vi "Set KH Coupling.vi"(8 "error in (no error)":errorcluster, 10 "Coupling":T1=enum."DC", 11 "KH Cluster":T2) -> (0 "error out":errorcluster, 3 "KH Cluster out":T2)   [LabVIEW 2016, in "Control Experiment UI.lvclass"]
uses:
  Control Experiment UI.lvclass
  Typedefs/KH Cluster--Cluster.ctl
  <userlib>/LevyLab/Krohn Hite 7008/typedefs/SetAll-Cluster.ctl
  <userlib>/LevyLab/Krohn Hite 7008/typedefs/Channel-Enum.ctl
  <userlib>/LevyLab/Krohn Hite 7008/typedefs/Gain-Enum.ctl
  <userlib>/LevyLab/Krohn Hite 7008/typedefs/Filter-Enum.ctl
  <userlib>/LevyLab/Krohn Hite 7008/typedefs/Shunt-Enum.ctl
  <userlib>/LevyLab/Krohn Hite 7008/typedefs/Coupling-Enum.ctl
  <userlib>/LevyLab/Krohn Hite 7008/typedefs/Input Configuration-Enum.ctl
  <userlib>/LevyLab/Krohn Hite 7008/Instrument.KH7008.lvclass
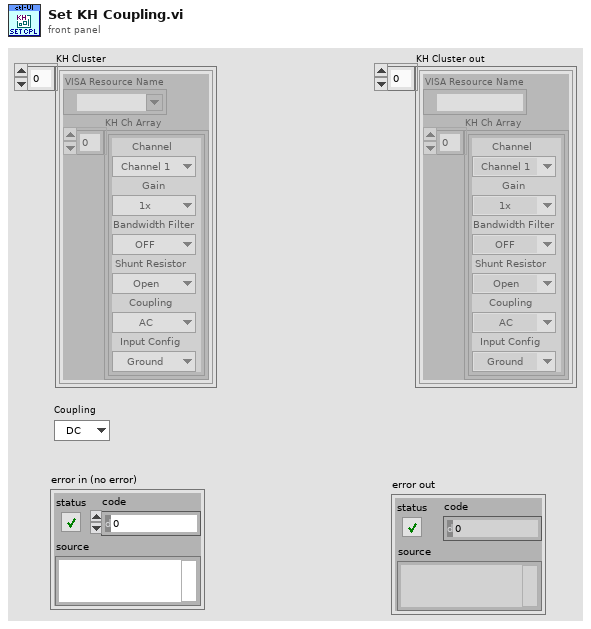
[diagram p1: front panel]
types:
  T1 = typedef "Instrument.KH7008.lvclass/Coupling-Enum.ctl" = enum16{"AC", "DC"}
  T2 = typedef "KH Cluster--Cluster.ctl" = cluster{"VISA Resource Name":refnum<visa-resource-name>, "KH Ch Array":T3[]}[]
  T3 = typedef "Instrument.KH7008.lvclass/SetAll-Cluster.ctl" = cluster{"Channel":T4, "Gain":T5, "Bandwidth Filter":T6, "Shunt Resistor":T7, "Coupling":T1, "Input Config":T8}
  T4 = typedef "Instrument.KH7008.lvclass/Channel-Enum.ctl" = enum16{"Channel 1", "Channel 2", "Channel 3", "Channel 4", "Channel 5", "Channel 6", "Channel 7", "Channel 8"}
  T5 = typedef "Instrument.KH7008.lvclass/Gain-Enum.ctl" = enum16{"1x", "10x", "100x", "1000x"}
  T6 = typedef "Instrument.KH7008.lvclass/Filter-Enum.ctl" = enum16{"OFF", "ON"}
  T7 = typedef "Instrument.KH7008.lvclass/Shunt-Enum.ctl" = enum16{"Open", "50 Ohms", "500 Ohms", "5k Ohms", "50k Ohms", "10M Ohm"}
  T8 = typedef "Instrument.KH7008.lvclass/Input Configuration-Enum.ctl" = enum16{"Ground", "SE+ (-gnd)", "SE- (+gnd)", "Differential"}
  T9 = cluster{"VISA Resource Name":refnum<visa-resource-name>, "KH Ch Array":T3[]}
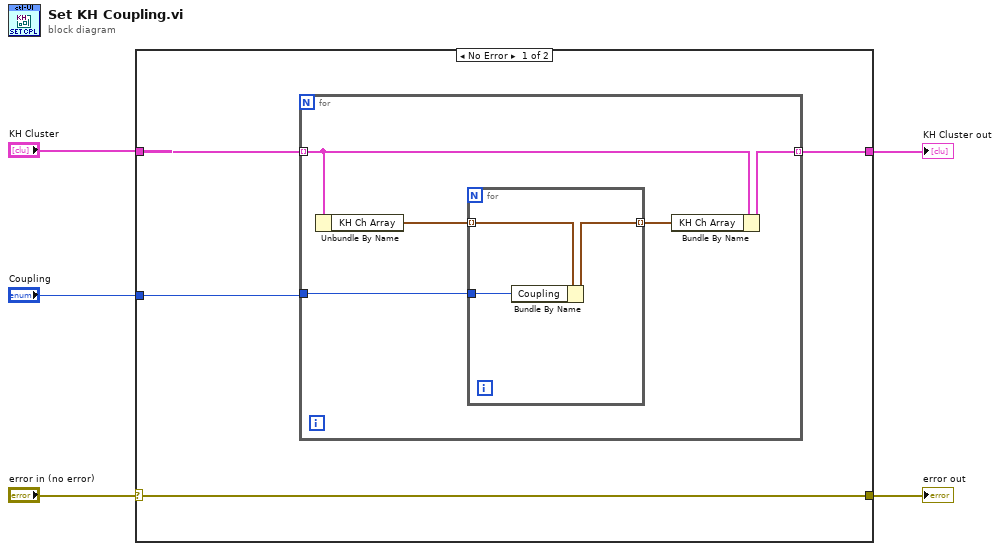
[diagram p0: block diagram]
diagram:
  n1 = case shown="No Error" "error in (no error)" {
    selector: "error in (no error)" -> [w8 w18]
    tunnel: "Coupling" -> [w6 _]
    tunnel: "KH Cluster" -> [w9 w19]
    tunnel: [w8 w18] -> w1
    tunnel: [w7 w19] -> w2
    frame No Error {
      n2 = for {
        tunnel: w9 -> [w14] mode=indexing
        tunnel: [w13] -> w7 mode=indexing
        tunnel: w6 -> [w10]
        n3 = Unbundle By Name(w14) -> ("KH Ch Array"=w12:T3[])
        n4 = for {
          tunnel: w12 -> [w17] mode=indexing
          tunnel: [w16] -> w11 mode=indexing
          tunnel: w10 -> [w15]
          n5 = Bundle By Name(cluster=w17, "Coupling"=w15) -> (w16:T3)
        }
        n6 = Bundle By Name(cluster=w14, "KH Ch Array"=w11) -> (w13:T9)
      }
    }
    frame Error {
    }
  }
  "KH Cluster out" <- w2
  "error out" <- w1
